vi "S to ABCD - 2nPort.vi"(8 "error in (no error)":errorcluster, 10 "Zc (Ohm)":cdb[](array[numeric]), 11 "S-par Array In":cdb[][](array[numeric])) -> (0 "error out":errorcluster, 3 "ABCD Array Out":cdb[][](array[numeric]))   [LabVIEW 2023, in "NI_HFNetworkAnalysis.lvlib"]
doc: "Convert a 2N-port S-parameter array to an ABCD array, where the characteristic impedance Zc is specified for each port:\n<b>{ v3, i3, v4, i4 } = ABCD . { v1, i1, v2, i2 }</b>\n\nInput S-parameter array rows are defined as <b>(S11,S12,S13,S14,...,S21,S22,S23,S24,...,S31,S32,S33,S34,...,S41,S42,S43,S44,...)</b>\nand output ABCD array rows are defined as <b>(a11,a12,a13,a14,...,a21,a22,a23,a24,...,a31,a32,a33,a34,...,a41,a42,a43,a44,...)</b>.\n\n<b>Note</b>\nThe convention for both S-parameters and ABCD arrays for the current is <b>\"positive when flowing into the port\"</b>.\n\n<b>Known Limitations</b>\nTransformation supports only 2n-port networks."
uses:
  NI_HFNetworkAnalysis.lvlib
  <vilib>/Analysis/baseanly.llb/Complex A x B.vi
  <vilib>/Analysis/Matrix/Numeric/Conversions/Array To Matrix - CA2.vi
  <vilib>/Analysis/baseanly.llb/Complex Inverse Matrix.vi
  <vilib>/Analysis/Matrix/Numeric/Conversions/Matrix To Array - CM.vi
  <vilib>/Analysis/Matrix/NI_Matrix.lvlib
  <vilib>/Analysis/NI_AALBase.lvlib
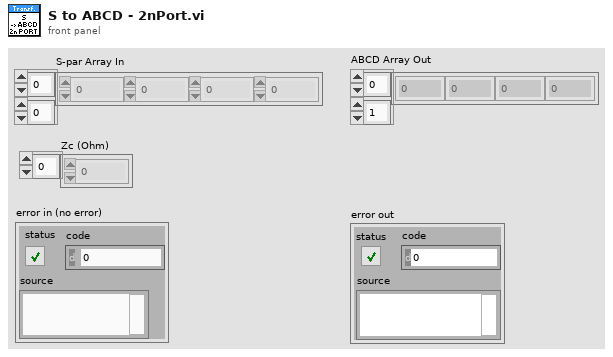
[diagram p1: front panel]
types:
  T1 = typedef "NI_Matrix.lvlib/ComplexMatrix.ctl" = cdb[][]
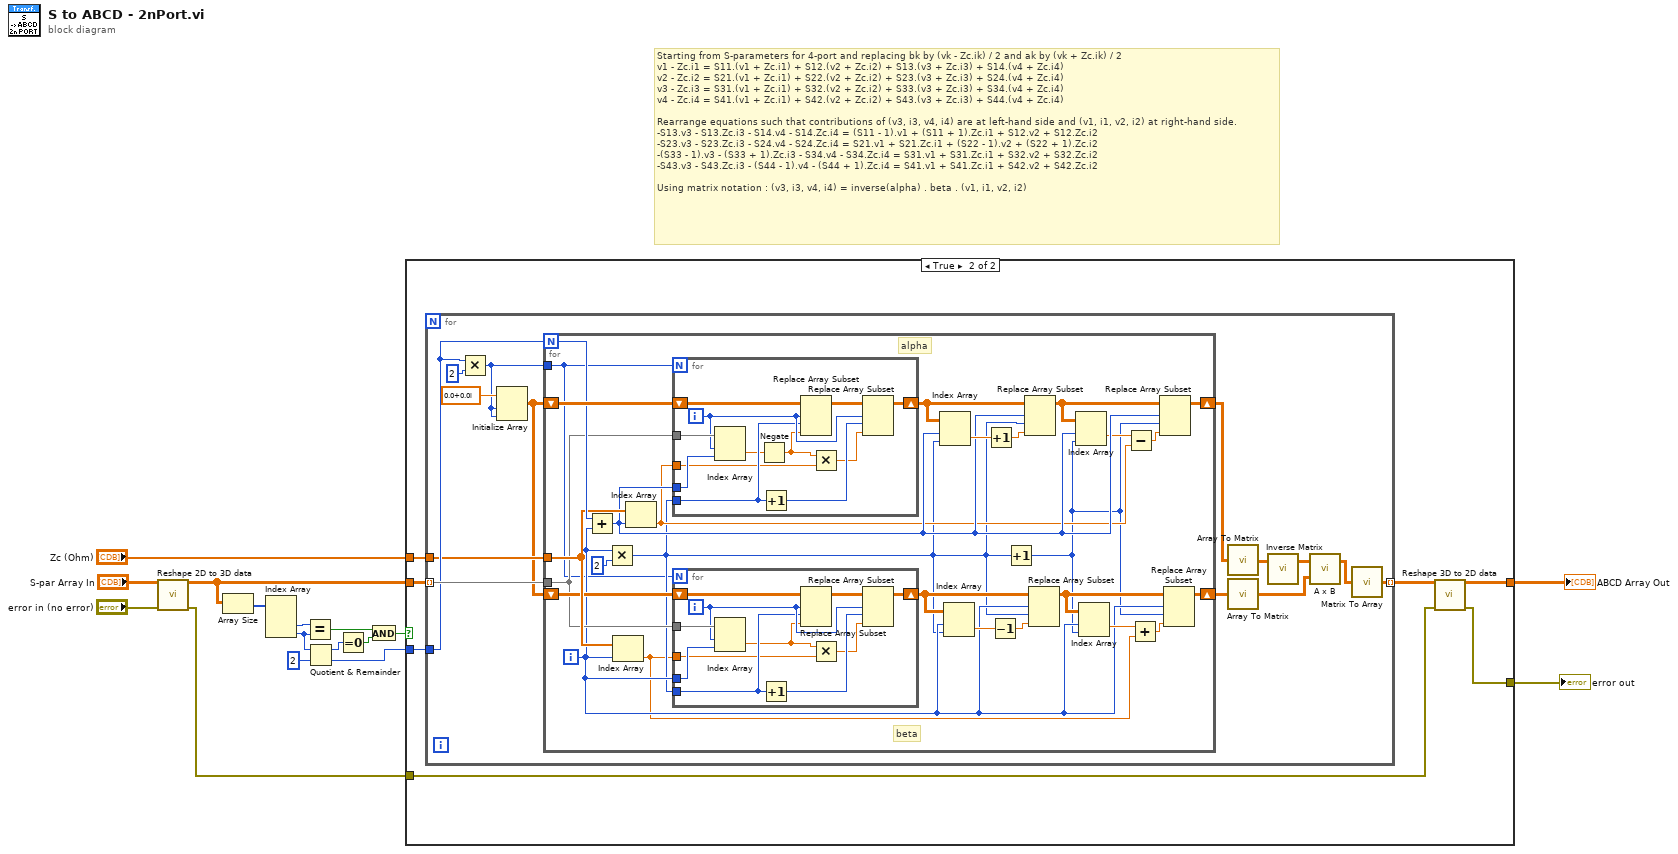
[diagram p0: block diagram]
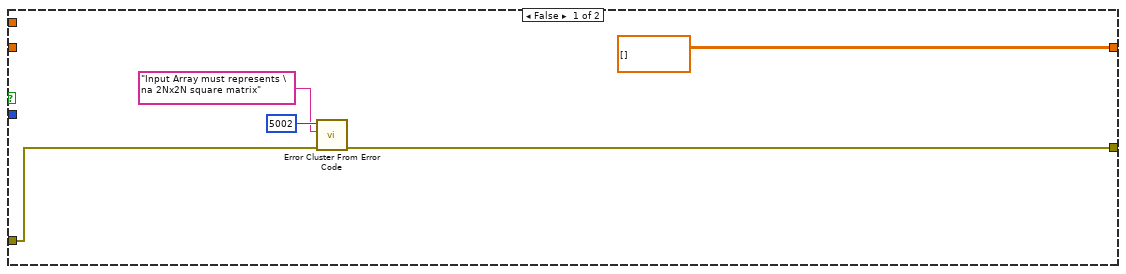
[diagram p2: hidden frame]
diagram:
  # "Starting from S-parameters for 4-port and replacing bk by (vk - Zc.ik) / 2 and ak by (vk + Zc.ik) / 2\nv1 - Zc.i1 = S11.(v1 + Zc.i1) + S12.(v2 + Zc.i2) + S13.(v3 + Zc.i3) + S14.(v4 + Zc.i4)\nv2 - Zc.i2 = S21.(v1 + Zc.i1) + S22.(v2 + Zc.i2) + S23.(v3 + Zc.i3) + S24.(v4 + Zc.i4)\nv3 - Zc.i3 = S31.(v1 + Zc.i1) + S32.(v2 + Zc.i2) + S33.(v3 + Zc.i3) + S34.(v4 + Zc.i4)\nv4 - Zc.i4 = S41.(v1 + Zc.i1) + S42.(v2 + Zc.i2) + S43.(v3 + Zc.i3) + S44.(v4 + Zc.i4)\n\nRearrange equations such that contributions of (v3, i3, v4, i4) are at left-hand side and (v1, i1, v2, i2) at right-hand side.\n-S13.v3 - S13.Zc.i3 - S14.v4 - S14.Zc.i4 = (S11 - 1).v1 + (S11 + 1).Zc.i1 + S12.v2 + S12.Zc.i2\n-S23.v3 - S23.Zc.i3 - S24.v4 - S24.Zc.i4 = S21.v1 + S21.Zc.i1 + (S22 - 1).v2 + (S22 + 1).Zc.i2\n-(S33 - 1).v3 - (S33 + 1).Zc.i3 - S34.v4 - S34.Zc.i4 = S31.v1 + S31.Zc.i1 + S32.v2 + S32.Zc.i2\n-S43.v3 - S43.Zc.i3 - (S44 - 1).v4 - (S44 + 1).Zc.i4 = S41.v1 + S41.Zc.i1 + S42.v2 + S42.Zc.i2\n\nUsing matrix notation : (v3, i3, v4, i4) = inverse(alpha) . beta . (v1, i1, v2, i2)"
  n1 = call "Reshape 2D to 3D data.vi"("Parameters In (2D)"="S-par Array In", "Error In"="error in (no error)") -> ("Parameters Out (3D)"=w15:cdb[][][], "Error Out"=w7:errorcluster)  [unwired: 12 in]
  n2 = Array Size(array=w15) -> (size(s)=w14:i32[])
  n3 = Index Array(array=w14) -> (element #2=w2:i32, element #3=w13:i32)  [unwired: 3 in, 1 out]
  n4 = Equal?(x=w2, y=w13) -> (x = y?=w11:bool)
  n5 = Quotient & Remainder(x=w13, y=2) -> (x-y*floor(x/y)=w4:i32, floor(x/y)=w3:i32)
  n6 = Equal To 0?(x=w4) -> (x = 0?=w10:bool)
  n7 = And(x=w11, y=w10) -> (x .and. y?=w9:bool)
  n8 = case shown="True" w9 {
    tunnel: w15 -> [_ w28]
    tunnel: w3 -> [_ w27]
    tunnel: [cdb[][] [] ("Parameters Out (2D)") w26] -> w8
    tunnel: w7 -> [w20 w23]
    tunnel: [w19 w24] -> w5
    tunnel: "Zc (Ohm)" -> [_ w25]
    frame False {
      n9 = call <vilib>:"Error Cluster From Error Code.vi"("error in (no error)"=w20, "error message (\"\")"="Input Array must represents \na 2Nx2N square matrix" ("error message (\"\")"), "error code (0)"=5002) -> ("error out"=w19:errorcluster)  [unwired: 6 in]
    }
    frame True {
      n10 = for {
        tunnel: w28 -> [w42] mode=indexing
        tunnel: w27 -> [w40]
        tunnel: w25 -> [w37]
        tunnel: [w30] -> w22 mode=indexing
        n11 = Multiply(x=w40, y=2) -> (x*y=w38:i32)
        n12 = Initialize Array(cdb 0.0+0.0i ("element"), w38, w38) -> (w36:cdb[][])
        n13 = for {
          N: w40 -> [w67]
          tunnel: w42 -> [w64]
          shift-right: [w55] -> w35
          shift-left: w36 -> [w69]
          tunnel: w38 -> [w43]
          tunnel: w37 -> [w66]
          shift-right: [w44] -> w34
          shift-left: w36 -> [w65]
          i -> [w48]
          # "beta"
          # "alpha"
          n14 = Add(x=w67, y=w48) -> (x+y=w59:i32)
          n15 = Multiply(x=w48, y=2) -> (x*y=w47:i32)
          n16 = Index Array(array=w66, index=w48) -> (element=w45:cdb)
          n17 = Index Array(array=w66, index=w59) -> (element=w56:cdb)
          n18 = for {
            N: w43 -> [_]
            shift-right: [w85] -> w63
            shift-left: w69 -> [w90]
            tunnel: w59 -> [w92]
            tunnel: w47 -> [w87]
            tunnel: w64 -> [w91]
            tunnel: w56 -> [w82]
            i -> [w88]
            n19 = Index Array(array=w91, index (row)=w88, index (col)=w92) -> (element=w84:cdb)
            n20 = Negate(x=w84) -> (-x=w83:cdb)
            n21 = Increment(x=w87) -> (x+1=w86:i32)
            n22 = Replace Array Subset(array=w90, new element=w83, index (row)=w88, index (col)=w87) -> (w89:cdb[][])
            n23 = Multiply(x=w83, y=w82) -> (x*y=w81:cdb)
            n24 = Replace Array Subset(array=w89, new element=w81, index (row)=w88, index (col)=w86) -> (w85:cdb[][])
          }
          n25 = for {
            N: w43 -> [_]
            shift-right: [w73] -> w49
            shift-left: w65 -> [w78]
            tunnel: w48 -> [w80]
            tunnel: w47 -> [w75]
            tunnel: w64 -> [w79]
            tunnel: w45 -> [w72]
            i -> [w76]
            n26 = Index Array(array=w79, index (row)=w76, index (col)=w80) -> (element=w70:cdb)
            n27 = Increment(x=w75) -> (x+1=w74:i32)
            n28 = Replace Array Subset(array=w78, new element=w70, index (row)=w76, index (col)=w75) -> (w77:cdb[][])
            n29 = Multiply(x=w70, y=w72) -> (x*y=w71:cdb)
            n30 = Replace Array Subset(array=w77, new element=w71, index (row)=w76, index (col)=w74) -> (w73:cdb[][])
          }
          n31 = Index Array(array=w63, index (row)=w59, index (col)=w47) -> (element=w62:cdb)
          n32 = Index Array(array=w49, index (row)=w48, index (col)=w47) -> (element=w54:cdb)
          n33 = Increment(x=w62) -> (x+1=w61:cdb)
          n34 = Decrement(x=w54) -> (x-1=w53:cdb)
          n35 = Increment(x=w47) -> (x+1=w46:i32)
          n36 = Replace Array Subset(array=w63, new element=w61, index (row)=w59, index (col)=w47) -> (w60:cdb[][])
          n37 = Replace Array Subset(array=w49, new element=w53, index (row)=w48, index (col)=w47) -> (w52:cdb[][])
          n38 = Index Array(array=w60, index (row)=w59, index (col)=w46) -> (element=w57:cdb)
          n39 = Index Array(array=w52, index (row)=w48, index (col)=w46) -> (element=w50:cdb)
          n40 = Subtract(x=w57, y=w56) -> (x-y=w58:cdb)
          n41 = Add(x=w50, y=w45) -> (x+y=w51:cdb)
          n42 = Replace Array Subset(array=w60, new element=w58, index (row)=w59, index (col)=w46) -> (w55:cdb[][])
          n43 = Replace Array Subset(array=w52, new element=w51, index (row)=w48, index (col)=w46) -> (w44:cdb[][])
        }
        n44 = call-poly <vilib>:"Array To Matrix.vi"("Complex 2D Array"=w35) -> ("Complex Matrix"=w33:T1)
        n45 = call-poly <vilib>:"Array To Matrix.vi"("Complex 2D Array"=w34) -> ("Complex Matrix"=w31:T1)
        n46 = call-poly <vilib>:"Inverse Matrix.vi"("Input Matrix"=w33) -> ("Inverse Matrix"=w32:T1)  [unwired: 1 in, 1 out]
        n47 = call-poly <vilib>:"A x B.vi"("B"=w31, "A"=w32) -> ("A x B"=w29:T1)  [unwired: 1 out]
        n48 = call-poly <vilib>:"Matrix To Array.vi"("Complex Matrix"=w29) -> ("Complex 2D Array"=w30:cdb[][])
      }
      n49 = call "Reshape 3D to 2D data.vi"("Parameters In (3D)"=w22, "Error In"=w23) -> ("Parameters Out (2D)"=w26:cdb[][], "Error Out"=w24:errorcluster)  [unwired: 12 in]
    }
  }
  "ABCD Array Out" <- w8
  "error out" <- w5
